vi "Scouting Compiler.vi"() -> ()   [LabVIEW 2015]
uses:
  <vilib>/Utility/sysdir.llb/System Directory Type.ctl
panel:
  out "array averaged":string[][](array[string])
  out "array":string[][](array[string])
  in  "input cluster":T1
  out "output cluster":T1
  in  "Sort By":u16(ring) items=["Team Number", "Rating", "Number of High Goals", "Number of Low Goals"]
  # "Team Number"
  # "Lift Gate"
  # "Teeter Totter"
  # "Moat"
  # "Rampart"
  # "Drawbridge"
  # "Sally Port"
  # "Rock Wall"
  # "Rough Terrain"
  # "Low Bar"
  # "Auto High Goal"
  # "Auto Low Goal"
  # "Scale"
  # "High Goals"
  # "Low Goal"
  # "Autonomous"
  # "Up to Defense"
  # "Rating"
  # "Comment"
  # "Team Number"
  # "Lift Gate"
  # "Teeter Totter"
  # "Moat"
  # "Rampart"
  # "Drawbridge"
  # "Sally Port"
  # "Rock Wall"
  # "Rough Terrain"
  # "Low Bar"
  # "Auto High Goal"
  # "Auto Low Goal"
  # "Scale"
  # "High Goals"
  # "Low Goal"
  # "Autonomous"
  # "Up to Defense"
  # "Rating"
  # "Comment"
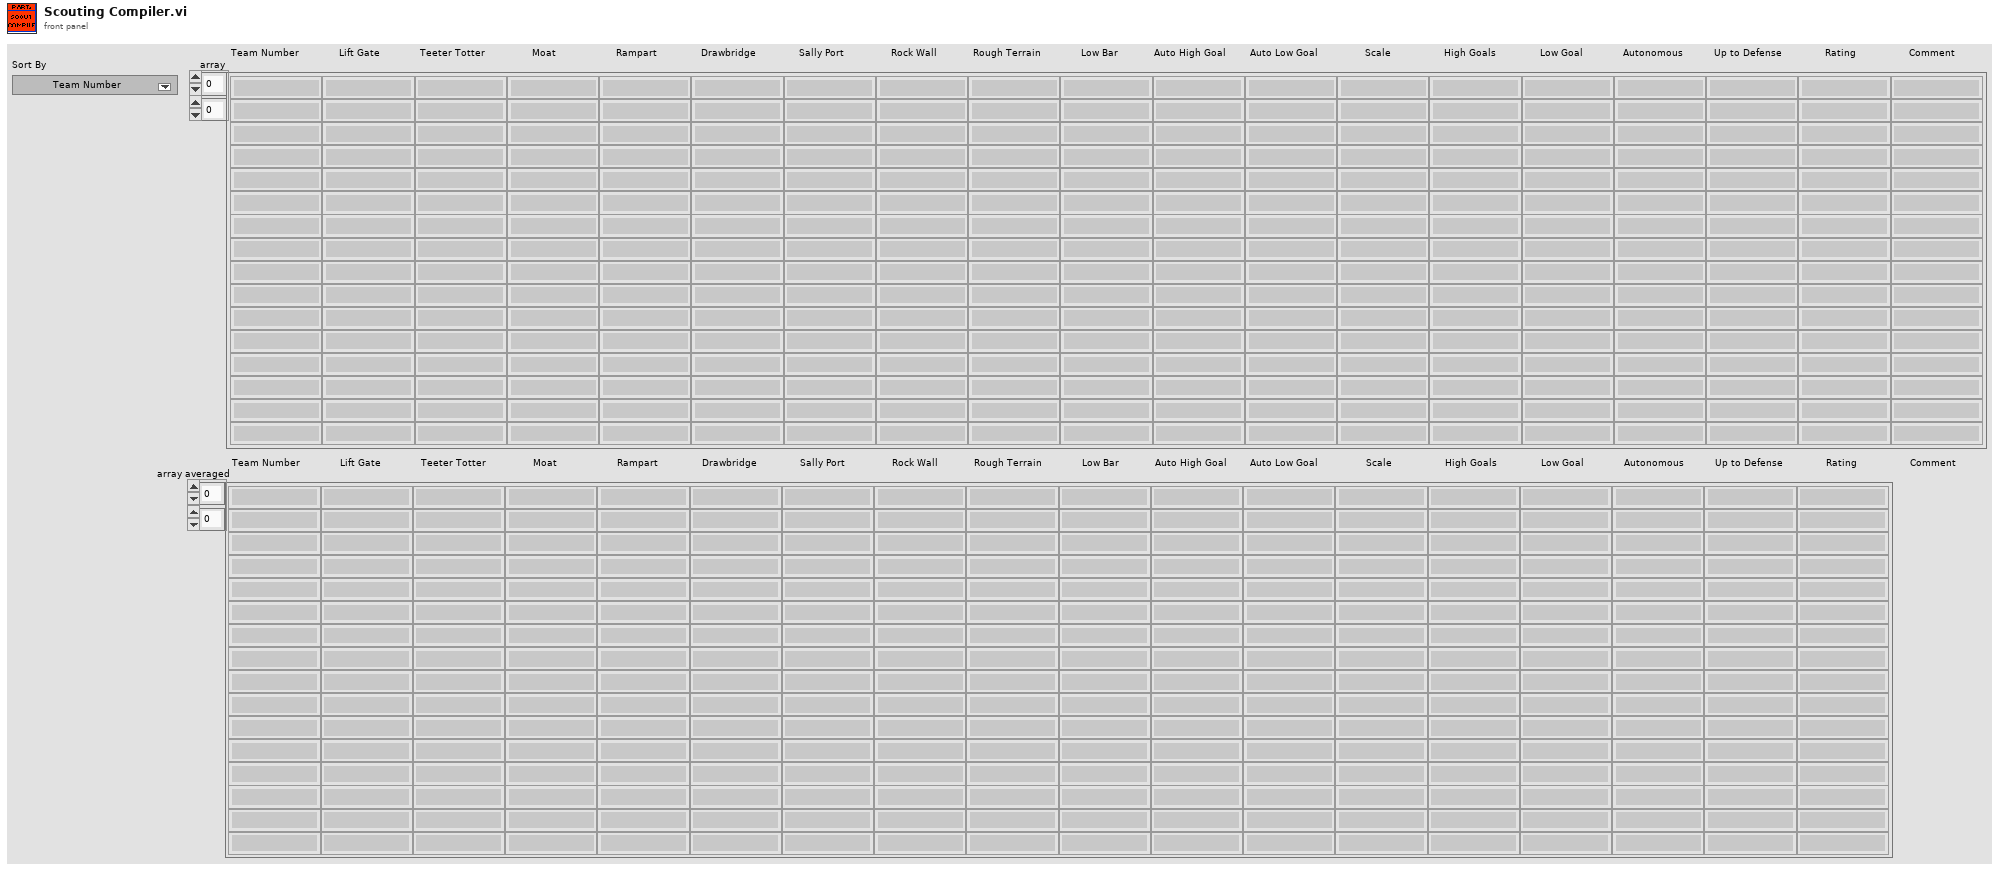
[diagram p1: front panel]
types:
  T1 = cluster{"String":string, "String 2":string, "String 3":string, "String 4":string, "String 5":string, "String 6":string, "String 7":string, "String 8":string, "String 9":string, "String 10":string, "String 11":string, "String 12":string, "String 13":string, "String 14":string, "String 15":string, "String 16":string, "String 17":string, "String 18":string}
  T2 = typedef "System Directory Type.ctl" = i32
  T3 = cluster{string, string, string, string, string, string, string, string, string, string, string, string, string, string, string, string, string, string, string}[]
  T4 = enum16{"open", "replace", "create", "open or create", "replace or create", "replace or create with confirmation"}
  T5 = cluster{"String":string, "String 2":string, "String 3":string, "String 4":string, "String 5":string, "String 6":string, "String 7":string, "String 8":string, "String 9":string, "String 10":string, "String 11":string, "String 12":string, "String 13":string, "String 14":string, "String 15":string, "String 16":string, "String 17":string, "String 18":string}[]
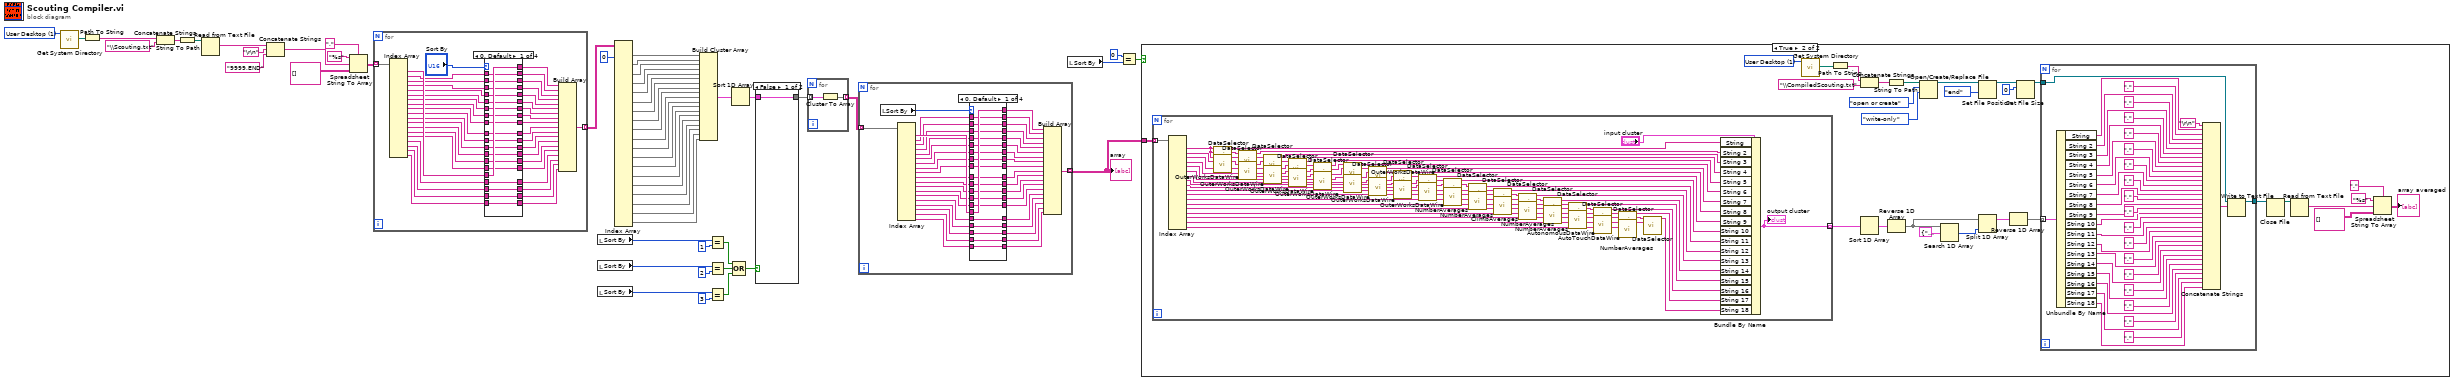
[diagram p0: block diagram]
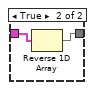
[diagram p6: hidden frame]
diagram:
  w49 = T2 1 items=["User Home"=0, "User Desktop"=1, "User Documents"=2, "User Application Data"=3, "User Preferences"=4, "User Temporary"=5, "Public Documents"=6, "Public Application Data"=7, "Public Preferences"=8, "Public Cache"=13, "System Core Libraries"=9, "System Installed Libraries"=10, "Application Files"=11, "Boot Volume Root"=12] ("system directory type")
  n1 = call <vilib>:"Get System Directory.vi"("system directory type"=w49) -> ("system directory"=w50:path)  [unwired: 10 in]
  n2 = Path To String(path=w50) -> (string=w51:string)
  n3 = Concatenate Strings(w51, "\\Scouting.txt" ("string")) -> (w53:string)
  n4 = String To Path(string=w53) -> (path=w48:path)
  n5 = Read from Text File(file (use dialog)=w48) -> (text=w4:string)  [unwired: 3 in, 3 out]
  n6 = Concatenate Strings(w4, "\r\n", "9999,END" ("string")) -> (w1:string)
  n7 = Spreadsheet String To Array(delimiter (Tab)=",", format string="%s", spreadsheet string=w1, array type (2D Dbl)=string[][] []) -> (array=w45:string[][])
  n8 = for {
    tunnel: w45 -> [w94] mode=indexing
    tunnel: [w57] -> w24 mode=indexing
    n9 = Index Array(array=w94) -> (element #1=w92:string, element #2=w90:string, element #3=w89:string, element #4=w86:string, element #5=w84:string, element #6=w82:string, element #7=w80:string, element #8=w78:string, element #9=w76:string, element #10=w74:string, element #11=w72:string, element #12=w70:string, element #13=w68:string, element #14=w66:string, element #15=w64:string, element #16=w62:string, element #17=w60:string, element #18=w58:string, element #19=w54:string)  [unwired: 19 in]
    n10 = case shown="0, Default" "Sort By" {
      tunnel: [w113 w131 w151 w153] -> w93
      tunnel: w92 -> [w113 w132 w150 w154]
      tunnel: [w112 w130 w149 w170] -> w91
      tunnel: w90 -> [w112 w130 w149 w170]
      tunnel: [w111 w129 w148 w169] -> w88
      tunnel: w89 -> [w111 w129 w148 w169]
      tunnel: [w110 w128 w147 w168] -> w87
      tunnel: w86 -> [w110 w128 w147 w168]
      tunnel: [w109 w127 w146 w167] -> w85
      tunnel: w84 -> [w109 w127 w146 w167]
      tunnel: [w108 w126 w145 w166] -> w83
      tunnel: w82 -> [w108 w126 w145 w166]
      tunnel: [w107 w125 w144 w165] -> w81
      tunnel: w80 -> [w107 w125 w144 w165]
      tunnel: [w106 w124 w143 w164] -> w79
      tunnel: w78 -> [w106 w124 w143 w164]
      tunnel: [w105 w123 w142 w163] -> w77
      tunnel: w76 -> [w105 w123 w142 w163]
      tunnel: [w104 w122 w141 w162] -> w75
      tunnel: w74 -> [w104 w122 w141 w162]
      tunnel: [w103 w121 w140 w161] -> w73
      tunnel: w72 -> [w103 w121 w140 w161]
      tunnel: [w102 w120 w139 w160] -> w71
      tunnel: w70 -> [w102 w120 w139 w160]
      tunnel: [w101 w119 w138 w159] -> w69
      tunnel: w68 -> [w101 w119 w138 w159]
      tunnel: [w100 w118 w150 w152] -> w67
      tunnel: w66 -> [w100 w118 w151 w152]
      tunnel: [w99 w117 w137 w154] -> w65
      tunnel: w64 -> [w99 w117 w137 w153]
      tunnel: [w98 w116 w136 w158] -> w63
      tunnel: w62 -> [w98 w116 w136 w158]
      tunnel: [w97 w115 w135 w157] -> w61
      tunnel: w60 -> [w97 w115 w135 w157]
      tunnel: [w96 w132 w134 w156] -> w59
      tunnel: w58 -> [w96 w131 w134 w156]
      tunnel: [w95 w114 w133 w155] -> w55
      tunnel: w54 -> [w95 w114 w133 w155]
      frame 0, Default {
      }
      frame 1 {
      }
      frame 2 {
      }
      frame 3 {
      }
    }
    n11 = Build Array(w93, w91, w88, w87, w85, w83, w81, w79, w77, w75, w73, w71, w69, w67, w65, w63, w61, w59, w55) -> (w57:string[])
  }
  n12 = local read "Sort By"() -> (w21:u16)
  n13 = local read "Sort By"() -> (w18:u16)
  n14 = local read "Sort By"() -> (w17:u16)
  n15 = Index Array(array=w24, index (col) #1=0 ("disabled index (col)")) -> (element #1=w44:string[], element #2=w43:string[], element #3=w42:string[], element #4=w41:string[], element #5=w40:string[], element #6=w39:string[], element #7=w38:string[], element #8=w37:string[], element #9=w36:string[], element #10=w35:string[], element #11=w34:string[], element #12=w33:string[], element #13=w32:string[], element #14=w31:string[], element #15=w30:string[], element #16=w29:string[], element #17=w28:string[], element #18=w27:string[], element #19=w25:string[])  [unwired: 37 in]
  n16 = Build Cluster Array ("Index & Bundle Cluster Array")(w44, w43, w42, w41, w40, w39, w38, w37, w36, w35, w34, w33, w32, w31, w30, w29, w28, w27, w25) -> (w26:T3)
  n17 = Equal?(x=w21, y=u16 1) -> (x = y?=w15:bool)
  n18 = Equal?(x=w18, y=u16 2) -> (x = y?=w14:bool)
  n19 = Equal?(x=w17, y=u16 3) -> (x = y?=w13:bool)
  n20 = Sort 1D Array(array=w26) -> (sorted array=w23:T3)
  n21 = Compound Arithmetic op=OR(w15, w14, w13) -> (w12:bool)
  n22 = case shown="False" w12 {
    tunnel: w23 -> [w171 w173]
    tunnel: [w171 w172] -> w22
    frame False {
    }
    frame True {
      n23 = Reverse 1D Array(array=w173) -> (reversed array=w172:T3)
    }
  }
  n24 = for {
    tunnel: w22 -> [w174] mode=indexing
    tunnel: [w175] -> w11 mode=indexing
    n25 = Cluster To Array(cluster=w174) -> (array=w175:string[])
  }
  n26 = for {
    tunnel: w11 -> [w216] mode=indexing
    tunnel: [w179] -> w9 mode=indexing
    n27 = local read "Sort By"() -> (w176:u16)
    n28 = Index Array(array=w216) -> (element #1=w214:string, element #2=w212:string, element #3=w211:string, element #4=w208:string, element #5=w206:string, element #6=w204:string, element #7=w202:string, element #8=w200:string, element #9=w198:string, element #10=w196:string, element #11=w194:string, element #12=w192:string, element #13=w190:string, element #14=w188:string, element #15=w186:string, element #16=w184:string, element #17=w182:string, element #18=w180:string, element #19=w177:string)  [unwired: 19 in]
    n29 = case shown="0, Default" w176 {
      tunnel: [w235 w253 w273 w275] -> w215
      tunnel: w214 -> [w235 w254 w272 w276]
      tunnel: [w234 w252 w271 w292] -> w213
      tunnel: w212 -> [w234 w252 w271 w292]
      tunnel: [w233 w251 w270 w291] -> w210
      tunnel: w211 -> [w233 w251 w270 w291]
      tunnel: [w232 w250 w269 w290] -> w209
      tunnel: w208 -> [w232 w250 w269 w290]
      tunnel: [w231 w249 w268 w289] -> w207
      tunnel: w206 -> [w231 w249 w268 w289]
      tunnel: [w230 w248 w267 w288] -> w205
      tunnel: w204 -> [w230 w248 w267 w288]
      tunnel: [w229 w247 w266 w287] -> w203
      tunnel: w202 -> [w229 w247 w266 w287]
      tunnel: [w228 w246 w265 w286] -> w201
      tunnel: w200 -> [w228 w246 w265 w286]
      tunnel: [w227 w245 w264 w285] -> w199
      tunnel: w198 -> [w227 w245 w264 w285]
      tunnel: [w226 w244 w263 w284] -> w197
      tunnel: w196 -> [w226 w244 w263 w284]
      tunnel: [w225 w243 w262 w283] -> w195
      tunnel: w194 -> [w225 w243 w262 w283]
      tunnel: [w224 w242 w261 w282] -> w193
      tunnel: w192 -> [w224 w242 w261 w282]
      tunnel: [w223 w241 w260 w281] -> w191
      tunnel: w190 -> [w223 w241 w260 w281]
      tunnel: [w222 w240 w272 w274] -> w189
      tunnel: w188 -> [w222 w240 w273 w274]
      tunnel: [w221 w239 w259 w276] -> w187
      tunnel: w186 -> [w221 w239 w259 w275]
      tunnel: [w220 w238 w258 w280] -> w185
      tunnel: w184 -> [w220 w238 w258 w280]
      tunnel: [w219 w237 w257 w279] -> w183
      tunnel: w182 -> [w219 w237 w257 w279]
      tunnel: [w218 w254 w256 w278] -> w181
      tunnel: w180 -> [w218 w253 w256 w278]
      tunnel: [w217 w236 w255 w277] -> w178
      tunnel: w177 -> [w217 w236 w255 w277]
      frame 0, Default {
      }
      frame 1 {
      }
      frame 2 {
      }
      frame 3 {
      }
    }
    n30 = Build Array(w215, w213, w210, w209, w207, w205, w203, w201, w199, w197, w195, w193, w191, w189, w187, w185, w183, w181, w178) -> (w179:string[])
  }
  "array" <- w9
  n31 = local read "Sort By"() -> (w7:u16)
  n32 = Equal?(x=u16 0, y=w7) -> (x = y?=w5:bool)
  n33 = case shown="True" w5 {
    tunnel: w9 -> [_ w314]
    frame False {
    }
    frame True {
      w309 = T2 1 items=["User Home"=0, "User Desktop"=1, "User Documents"=2, "User Application Data"=3, "User Preferences"=4, "User Temporary"=5, "Public Documents"=6, "Public Application Data"=7, "Public Preferences"=8, "Public Cache"=13, "System Core Libraries"=9, "System Installed Libraries"=10, "Application Files"=11, "Boot Volume Root"=12] ("system directory type")
      n34 = for {
        tunnel: w314 -> [w449] mode=indexing
        tunnel: [w448] -> w320 mode=indexing
        n35 = Index Array(array=w449) -> (element #1=w386:string, element #2=w385:string, element #3=w384:string, element #4=w383:string, element #5=w382:string, element #6=w381:string, element #7=w380:string, element #8=w379:string, element #9=w378:string, element #10=w377:string, element #11=w375:string, element #12=w373:string, element #13=w366:string, element #14=w365:string, element #15=w364:string, element #16=w363:string, element #17=w362:string, element #18=w361:string)  [unwired: 18 in]
        n36 = call "DataSelector.vi"("Number in"=w386, "String in"=w386) -> ("String out"=w443:string, "Number out"=w445:string)  [unwired: 12 in]
        n37 = call "OuterWorksDataWire.vi"("String in"=w385, "Number in"=w386) -> ("Number out"=w394:string, "String out"=w444:string)  [unwired: 8 in]
        n38 = call "DataSelector.vi"("Number in"=w445, "String in"=w444) -> ("String out"=w442:string, "Number out"=w441:string)  [unwired: 12 in]
        n39 = call "OuterWorksDataWire.vi"("String in"=w384, "Number in"=w394) -> ("Number out"=w393:string, "String out"=w440:string)  [unwired: 8 in]
        n40 = call "DataSelector.vi"("Number in"=w441, "String in"=w440) -> ("String out"=w446:string, "Number out"=w439:string)  [unwired: 12 in]
        n41 = call "OuterWorksDataWire.vi"("String in"=w383, "Number in"=w393) -> ("Number out"=w392:string, "String out"=w438:string)  [unwired: 8 in]
        n42 = call "DataSelector.vi"("Number in"=w439, "String in"=w438) -> ("String out"=w437:string, "Number out"=w436:string)  [unwired: 12 in]
        n43 = call "OuterWorksDataWire.vi"("String in"=w382, "Number in"=w392) -> ("Number out"=w391:string, "String out"=w435:string)  [unwired: 8 in]
        n44 = call "DataSelector.vi"("Number in"=w436, "String in"=w435) -> ("String out"=w434:string, "Number out"=w433:string)  [unwired: 12 in]
        n45 = call "OuterWorksDataWire.vi"("String in"=w381, "Number in"=w391) -> ("Number out"=w390:string, "String out"=w432:string)  [unwired: 8 in]
        n46 = call "DataSelector.vi"("Number in"=w433, "String in"=w432) -> ("String out"=w431:string, "Number out"=w430:string)  [unwired: 12 in]
        n47 = call "OuterWorksDataWire.vi"("String in"=w380, "Number in"=w390) -> ("Number out"=w389:string, "String out"=w429:string)  [unwired: 8 in]
        n48 = call "DataSelector.vi"("Number in"=w430, "String in"=w429) -> ("String out"=w428:string, "Number out"=w427:string)  [unwired: 12 in]
        n49 = call "OuterWorksDataWire.vi"("String in"=w379, "Number in"=w389) -> ("Number out"=w388:string, "String out"=w426:string)  [unwired: 8 in]
        n50 = call "DataSelector.vi"("Number in"=w427, "String in"=w426) -> ("String out"=w425:string, "Number out"=w424:string)  [unwired: 12 in]
        n51 = call "OuterWorksDataWire.vi"("String in"=w378, "Number in"=w388) -> ("Number out"=w387:string, "String out"=w423:string)  [unwired: 8 in]
        n52 = call "DataSelector.vi"("Number in"=w424, "String in"=w423) -> ("String out"=w422:string, "Number out"=w421:string)  [unwired: 12 in]
        n53 = call "OuterWorksDataWire.vi"("String in"=w377, "Number in"=w387) -> ("Number out"=w376:string, "String out"=w420:string)  [unwired: 8 in]
        n54 = call "DataSelector.vi"("Number in"=w421, "String in"=w420) -> ("String out"=w419:string, "Number out"=w418:string)  [unwired: 12 in]
        n55 = call "NumberAverages.vi"("Number in"=w376, "String in"=w375) -> ("String out"=w417:string, "Number out"=w374:string)  [unwired: 7 in]
        n56 = call "DataSelector.vi"("Number in"=w418, "String in"=w417) -> ("String out"=w416:string, "Number out"=w415:string)  [unwired: 12 in]
        n57 = call "NumberAverages.vi"("Number in"=w374, "String in"=w373) -> ("String out"=w414:string, "Number out"=w372:string)  [unwired: 7 in]
        n58 = call "DataSelector.vi"("Number in"=w415, "String in"=w414) -> ("String out"=w413:string, "Number out"=w412:string)  [unwired: 12 in]
        n59 = call "ClimbAverages.vi"("Number in"=w372, "String in"=w366) -> ("String out"=w411:string, "Number out"=w371:string)  [unwired: 7 in]
        n60 = call "DataSelector.vi"("Number in"=w412, "String in"=w411) -> ("String out"=w410:string, "Number out"=w409:string)  [unwired: 12 in]
        n61 = call "NumberAverages.vi"("Number in"=w371, "String in"=w365) -> ("String out"=w408:string, "Number out"=w370:string)  [unwired: 7 in]
        n62 = call "DataSelector.vi"("Number in"=w409, "String in"=w408) -> ("String out"=w407:string, "Number out"=w406:string)  [unwired: 12 in]
        n63 = call "NumberAverages.vi"("Number in"=w370, "String in"=w364) -> ("String out"=w405:string, "Number out"=w369:string)  [unwired: 7 in]
        n64 = call "DataSelector.vi"("Number in"=w406, "String in"=w405) -> ("String out"=w404:string, "Number out"=w403:string)  [unwired: 12 in]
        n65 = call "AutonomousDataWire.vi"("String in"=w363, "Number in"=w369) -> ("Number out"=w368:string, "String out"=w402:string)  [unwired: 8 in]
        n66 = call "DataSelector.vi"("Number in"=w403, "String in"=w402) -> ("String out"=w401:string, "Number out"=w400:string)  [unwired: 12 in]
        n67 = call "AutoTouchDataWire.vi"("String in"=w362, "Number in"=w368) -> ("Number out"=w367:string, "String out"=w399:string)  [unwired: 8 in]
        n68 = call "DataSelector.vi"("Number in"=w400, "String in"=w399) -> ("String out"=w398:string, "Number out"=w397:string)  [unwired: 12 in]
        n69 = call "NumberAverages.vi"("Number in"=w367, "String in"=w361) -> ("String out"=w395:string)  [unwired: 7 in, 1 out]
        n70 = call "DataSelector.vi"("Number in"=w397, "String in"=w395) -> ("String out"=w396:string)  [unwired: 12 in, 1 out]
        n71 = Bundle By Name(cluster="input cluster", "String"=w443, "String 2"=w442, "String 3"=w446, "String 4"=w437, "String 5"=w434, "String 6"=w431, "String 7"=w428, "String 8"=w425, "String 9"=w422, "String 10"=w419, "String 11"=w416, "String 12"=w413, "String 13"=w410, "String 14"=w407, "String 15"=w404, "String 16"=w401, "String 17"=w398, "String 18"=w396) -> (w448:T1)
        "output cluster" <- w448
      }
      n72 = call <vilib>:"Get System Directory.vi"("system directory type"=w309) -> ("system directory"=w308:path)  [unwired: 10 in]
      n73 = Path To String(path=w308) -> (string=w307:string)
      n74 = Concatenate Strings(w307, "\\CompiledScouting.txt" ("string")) -> (w305:string)
      n75 = Sort 1D Array(array=w320) -> (sorted array=w319:T5)
      n76 = String To Path(string=w305) -> (path=w304:path)
      n77 = Reverse 1D Array(array=w319) -> (reversed array=w316:T5)
      n78 = Open/Create/Replace File(file path (use dialog)=w304, operation (0:open)=T4."open or create", access (0:read/write)=enum16{"read/write", "read-only", "write-only"}."write-only") -> (refnum out=w311:refnum<file>)  [unwired: 3 in, 2 out]
      n79 = Search 1D Array(1D array=w316, element=T1 {"String"="", "String 2"="", "String 3"="", "String 4"="", "String 5"="", "String 6"="", "String 7"="", "String 8"="", "String 9"="", "String 10"="", "String 11"="", "String 12"="", "String 13"="", "String 14"="", "String 15"="", "String 16"="", "String 17"="", "String 18"=""}) -> (index of element=w317:i32)  [unwired: 1 in]
      n80 = Set File Position(refnum=w311, from (0:start)=enum16{"start", "end", "current"}."end") -> (refnum out=w296:refnum<file>)  [unwired: 2 in, 1 out]
      n81 = Split 1D Array(array=w316, index=w317) -> (first subarray=w315:T5)  [unwired: 1 out]
      n82 = Reverse 1D Array(array=w315) -> (reversed array=w303:T5)
      n83 = Set File Size(6:i64 0 ("size (in bytes)"), 7:w296) -> (3:w294:refnum<file>)  [unwired: 1 in, 1 out]
      n84 = for {
        tunnel: w303 -> [w360] mode=indexing
        tunnel: w294 -> [w322]
        tunnel: [w321] -> w302
        n85 = Unbundle By Name(w360) -> ("String"=w359:string, "String 2"=w357:string, "String 3"=w355:string, "String 4"=w353:string, "String 5"=w351:string, "String 6"=w349:string, "String 7"=w347:string, "String 8"=w345:string, "String 9"=w343:string, "String 10"=w341:string, "String 11"=w339:string, "String 12"=w337:string, "String 13"=w335:string, "String 14"=w333:string, "String 15"=w331:string, "String 16"=w329:string, "String 17"=w327:string, "String 18"=w325:string)
        n86 = Concatenate Strings("\r\n", w359, "," ("string"), w357, "," ("string"), w355, "," ("string"), w353, "," ("string"), w351, "," ("string"), w349, "," ("string"), w347, "," ("string"), w345, "," ("string"), w343, "," ("string"), w341, "," ("string"), w339, "," ("string"), w337, "," ("string"), w335, "," ("string"), w333, "," ("string"), w331, "," ("string"), w329, "," ("string"), w327, "," ("string"), w325) -> (w323:string)
        n87 = Write to Text File(file (use dialog)=w322, text=w323) -> (refnum out=w321:refnum<file>)  [unwired: 2 in, 2 out]
      }
      n88 = Close File(refnum=w302) -> (path=w298:path)  [unwired: 1 in, 1 out]
      n89 = Read from Text File(file (use dialog)=w298) -> (text=w299:string)  [unwired: 3 in, 3 out]
      n90 = Spreadsheet String To Array(delimiter (Tab)=",", format string="%s", spreadsheet string=w299, array type (2D Dbl)=string[][] []) -> (array=→"array averaged":string[][])
    }
  }
